vi "ziImpedanceCalibInterp.vi"(2 "Frequencies (Hz)":dbl[](array[numeric]), 3 "Measurement_Z (F,X0,Y0,...Xn,Yn)":dbl[][](array[numeric])) -> (0 "Extrapolated":bool, 1 "Interpolated_Z (Series,F)":cdb[][](array[numeric]))   [LabVIEW 2018, in "Zurich Instruments LabOne.lvlib"]
doc: "Interpolates the calibration impedance to the frequency axis of the current measurement.\n<B>Frequencies (Hz)</B> is a sorted, ascending list of values frequencies."
uses:
  Zurich Instruments LabOne.lvlib
  <vilib>/gmath/NI_Gmath.lvlib
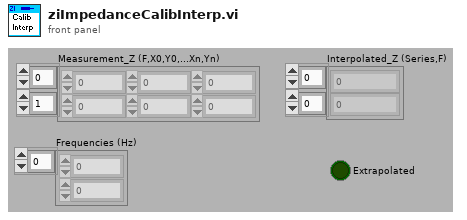
[diagram p1: front panel]
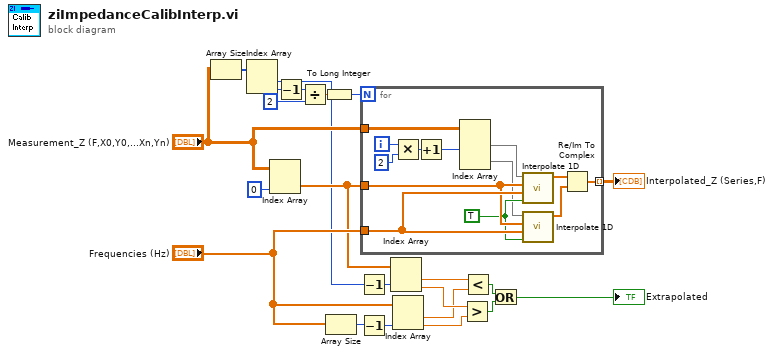
[diagram p0: block diagram]
diagram:
  n1 = Array Size(array="Measurement_Z (F,X0,Y0,...Xn,Yn)") -> (size(s)=w7:i32[])
  n2 = Index Array(array=w7) -> (element #1=w5:i32, element #2=w6:i32)  [unwired: 2 in]
  n3 = Index Array(array="Measurement_Z (F,X0,Y0,...Xn,Yn)", index (col)=0 ("index (row)")) -> (element=w17:dbl[])  [unwired: 1 in]
  n4 = Decrement(x=w6) -> (x-1=w1:i32)
  n5 = Divide(x=w1, y=2) -> (x/y=w4:dbl)
  n6 = To Long Integer(number=w4) -> (32bit integer=w2:i32)
  n7 = Array Size(array="Frequencies (Hz)") -> (size(s)=w19:i32)
  n8 = Decrement(x=w5) -> (x-1=w16:i32)
  n9 = Decrement(x=w19) -> (x-1=w18:i32)
  n10 = for {
    N: w2 -> [_]
    tunnel: [w33] -> w21 mode=indexing
    tunnel: "Frequencies (Hz)" -> [w32]
    tunnel: w17 -> [w31]
    tunnel: "Measurement_Z (F,X0,Y0,...Xn,Yn)" -> [w29]
    i -> [w28]
    w30 = TRUE ("X is monotonic")
    n11 = Multiply(x=w28, y=2) -> (x*y=w26:i32)
    n12 = Increment(x=w26) -> (x+1=w23:i32)
    n13 = Index Array(array=w29, index (col) #1=w23) -> (element #1=w25:dbl[], element #2=w24:dbl[])  [unwired: 3 in]
    n14 = call <vilib>:"Interpolate 1D.vi"("X is monotonic"=w30, "xi"=w32, "X"=w31, "Y"=w25) -> ("yi"=w34:dbl[])  [unwired: 5 in, 2 out]
    n15 = call <vilib>:"Interpolate 1D.vi"("X is monotonic"=w30, "xi"=w32, "X"=w31, "Y"=w24) -> ("yi"=w35:dbl[])  [unwired: 5 in, 2 out]
    n16 = Re/Im To Complex(1:w35, 2:w34) -> (0:w33:cdb[])
  }
  "Interpolated_Z (Series,F)" <- w21
  n17 = Index Array(array=w17, index #2=w16) -> (element #1=w13:dbl, element #2=w15:dbl)  [unwired: 1 in]
  n18 = Index Array(array="Frequencies (Hz)", index #2=w18) -> (element #1=w12:dbl, element #2=w14:dbl)  [unwired: 1 in]
  n19 = Greater?(x=w15, y=w14) -> (0:w10:bool)
  n20 = Less?(x=w13, y=w12) -> (x < y?=w11:bool)
  n21 = Or(x=w11, y=w10) -> (x .or. y?=→"Extrapolated":bool)
